vi "Channel_ToEasyObj.vi"(8 "error in (no error)":errorcluster, 11 "Channel in":refnum<class "Channel.lvclass">) -> (0 "error out":errorcluster, 2 "output cluster":T1 {"Data Reference" format="%.0x"}, 3 "Channel out":refnum<class "Channel.lvclass">)   [LabVIEW 2023, in "Channel.lvclass"]
doc: "Convert the class data into a cluster definition. Used for transferring the definitions between the System Explorer and the Engine."
uses:
  Channel.lvclass
  ChannelAsCluster.ctl
  <vilib>/NI VeriStand/Custom Device API/Data Reference.ctl
  Meta Data.ctl
  Channel.lvclass/Channel.ctl
  <vilib>/NI VeriStand/Custom Device API/Custom Device API.lvlib
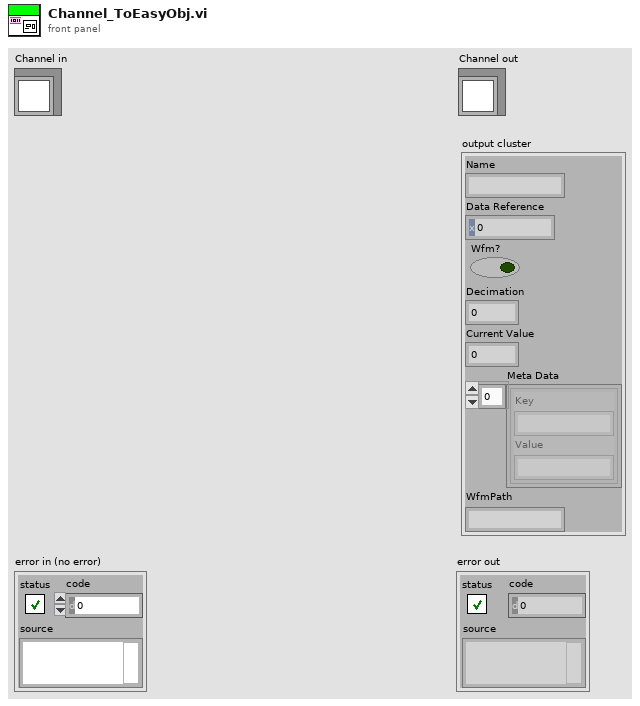
[diagram p1: front panel]
types:
  T1 = typedef "ChannelAsCluster.ctl" = cluster{"Name":string, "Data Reference":T2, "Wfm?":bool, "Decimation":i32, "Current Value":dbl, "Meta Data":T3[], "WfmPath":string}
  T2 = typedef "Custom Device API.lvlib/Data Reference.ctl" = i32
  T3 = typedef "Meta Data.ctl" = cluster{"Key":string, "Value":string}
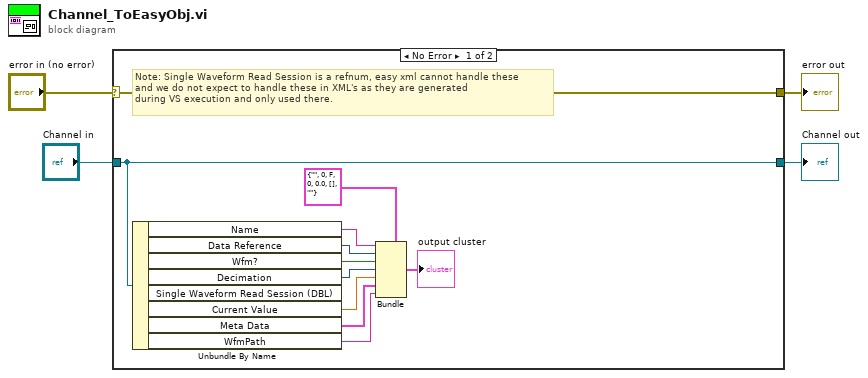
[diagram p0: block diagram]
diagram:
  n1 = case shown="No Error" "error in (no error)" {
    selector: "error in (no error)" -> [w15 w17]
    tunnel: [w15 w17] -> w3
    tunnel: [w10 w16] -> w1
    tunnel: "Channel in" -> [w10 w16]
    frame No Error {
      # "Note: Single Waveform Read Session is a refnum, easy xml cannot handle these\nand we do not expect to handle these in XML's as they are generated\nduring VS execution and only used there."
      n2 = Unbundle By Name(w10) -> ("Name"=w14:string, "Data Reference"=w13:T2, "Wfm?"=w12:bool, "Decimation"=w8:i32, "Current Value"=w7:dbl, "Meta Data"=w6:T3[], "WfmPath"=w5:string)  [unwired: 1 out]
      n3 = Bundle(cluster=T1 {"Name"="", "Data Reference"=0, "Wfm?"=FALSE, "Decimation"=0, "Current Value"=0.0, "Meta Data"=[], "WfmPath"=""} ("output cluster"), "Name"=w14, "Data Reference"=w13, "Wfm?"=w12, "Decimation"=w8, "Current Value"=w7, "Meta Data"=w6, "WfmPath"=w5) -> (→"output cluster":T1)
    }
    frame Error {
    }
  }
  "error out" <- w3
  "Channel out" <- w1
